vi "genIOL_Aligning.vi"(0 "Iris path":path=path "D:/IRISSoft LV2016 beta/Host Demo/ThorlabsData/Eye1/VSCAN_0002.raw", 1 "endJ5":dbl=30000.0, 2 "PC path":path=path "D:/IRISSoft LV2016 beta/Host Demo/ThorlabsData/Eye1/VSCAN_0003.raw", 3 "endPt":dbl[](array[numeric]), 4 "Distance from incision":dbl=1.0, 5 "OCT offset":dbl=13.0) -> (6 "Align_traj":dbl[][](array[numeric]), 7 "Inject_traj":dbl[][](array[numeric]), 8 "Whole_traj":dbl[][](array[numeric]))   [LabVIEW 2016]
uses:
  <vilib>/Math Plots/3D Math Plots/3D Scatter/3D Scatter XCtrl/3D Scatter.xctl
  Subsystems/Global Variables.vi
  <vilib>/Utility/file.llb/Write Delimited Spreadsheet (DBL).vi
  <vilib>/Math Plots/3D Math Plots/3D Scatter/3D Scatter Datatype/Public/Plot Helper (Vector).vi
  <vilib>/Analysis/NI_AALBase.lvlib
  <vilib>/Analysis/1siggen.llb/Ramp Pattern by Samples.vi
  <vilib>/gmath/NI_Gmath.lvlib
  <vilib>/Math Plots/3D Math Plots/3D Scatter/3D Scatter Datatype/3D Scatter Datatype.lvclass
  <vilib>/Math Plots/3D Math Plots/3D Plot/3D Plot Datatype/3D Plot Datatype.lvclass
panel:
  out "Actual Injection Plot 2":refnum<class "3D Plot Datatype.lvclass">[](xcontrol)
  out "current loop # 3":dbl
  out "Actual joint angles":dbl[][](array[numeric])
  out "Planned joint angles":dbl[][](array[numeric])
  out "Planned injection":dbl[][](array[numeric])
  out "Incision point index 3":dbl
  out "Incision point index 2":dbl
  out "Error in operational space":dbl[][](graph)
  out "current loop # 2":dbl
  out "time":dbl[](array[numeric])
  out "incision":dbl[](array[numeric])
  out "traj operational space":dbl[][](array[numeric])
  out "Incision point":dbl[](array[numeric])
  out "Implement Injection Plot":refnum<class "3D Plot Datatype.lvclass">[](xcontrol)
  out "Implement joint angles":dbl[][](graph)
  out "min dist":dbl
  out "Actual Injection Plot":refnum<class "3D Plot Datatype.lvclass">[](xcontrol)
  out "End manual joint":dbl[](array[numeric])
  out "Start manual joint":dbl[](array[numeric])
  out "Planed joint angles":dbl[][](graph)
  out "Actual joint angles":dbl[][](graph)
  out "traj":dbl[][](array[numeric])
  out "max dist":dbl
  out "Offset":dbl[][](array[numeric])
  out "Incision point index":dbl
  out "Planed Injection Plot":refnum<class "3D Plot Datatype.lvclass">[](xcontrol)
  out "current loop #":dbl
  out "x coordinates size 3":dbl
  out "x coordinates size 2":dbl
  out "x coordinates size":dbl
  out "x coordinates":dbl[](array[numeric])
  out "z coordinates":dbl[](array[numeric]) format="%#_13g"
  out "y coordinates":dbl[](array[numeric]) format="%#_13g"
  out "x coodi 2nd":dbl[](array[numeric]) format="%#_13g"
  in  "Total Time":dbl=60.0
  in  "Arm ID Ind":i32
  in  "Tip out Posit":dbl[](array[numeric])=[0.0, 0.0, 0.0] caption="Position [mm]" format="%#.3f"
  in  "Cycle Time [sec]":dbl[](array[numeric])=[60.0, 90.0, 120.0]
  out "zVisTraj":dbl[](array[numeric]) format="%_6g"
  out "yVisTraj":dbl[](array[numeric]) format="%_6g"
  out "xVisTraj":dbl[](array[numeric]) format="%_6g"
  in  "Sampling Rate [Hz]":i32=1000
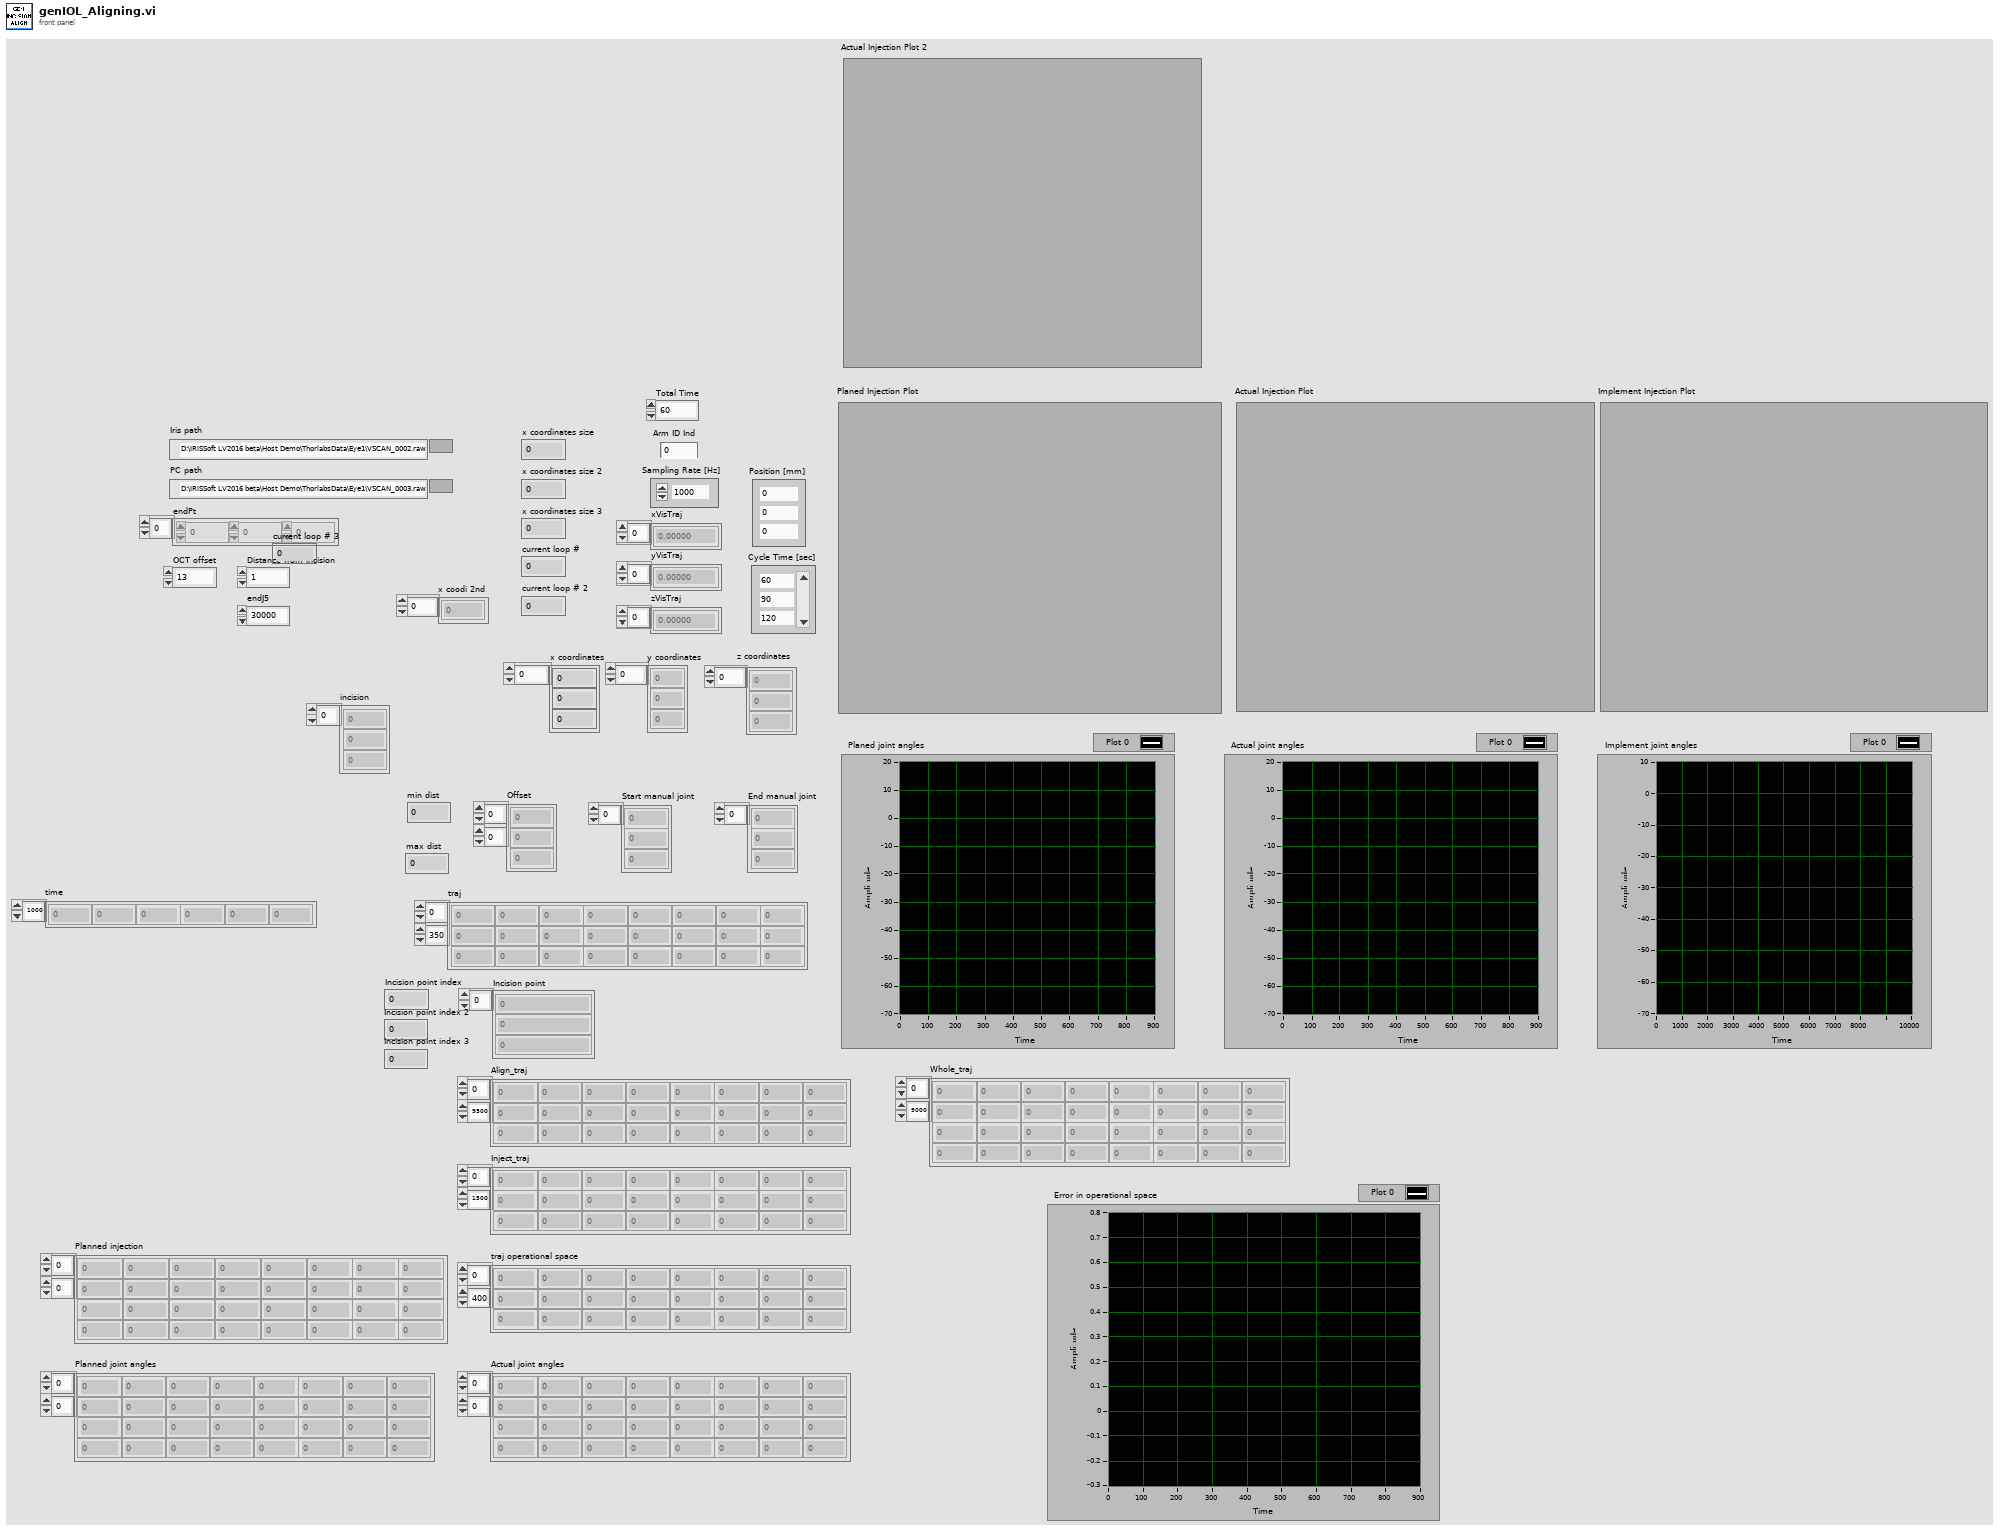
[diagram p1: front panel]
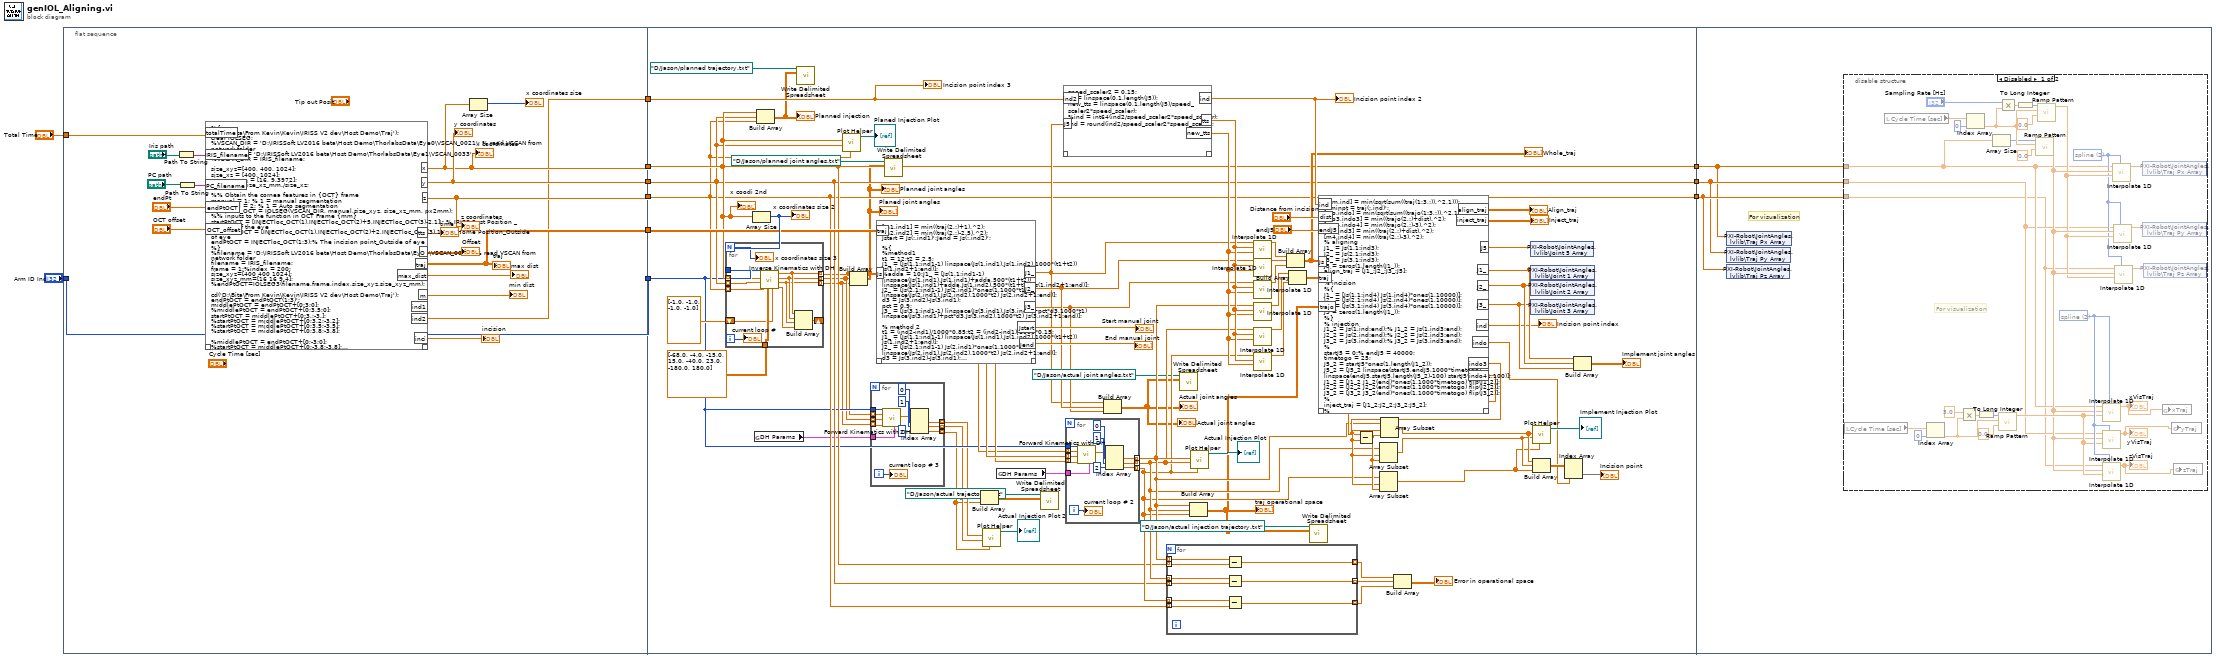
[diagram p0: block diagram]
diagram:
  n1 = flat-sequence {
    tunnel: "Arm ID Ind" -> [w30]
    tunnel: [w30] -> w10
    tunnel: [w26] -> w6
    tunnel: [w28] -> w5
    tunnel: [w27] -> w4
    tunnel: "Total Time" -> [w29]
    tunnel: [w13] -> w2
    tunnel: [w12] -> w1
    tunnel: w10 -> [w39]
    tunnel: [w52] -> w9
    tunnel: [w51] -> w8
    tunnel: [w50] -> w7
    tunnel: w6 -> [w52]
    tunnel: w5 -> [w51]
    tunnel: w4 -> [w50]
    tunnel: w2 -> [w63]
    tunnel: w1 -> [w54]
    tunnel: w9 -> [w152]
    tunnel: w8 -> [w153]
    tunnel: w7 -> [w154]
    frame #0 {
      n2 = Path To String(path="Iris path") -> (string=w20:string)
      n3 = Path To String(path="PC path") -> (string=w21:string)
      n4 = script code="%{\ncd('D:\\Bita\\From Kevin\\Kevin\\IRISS V2 dev\\Host Demo\\Traj');\nclear IOLSEG;\n%VSCAN_DIR = 'D:\\IRISSoft LV2016 beta\\Host Demo\\ThorlabsData\\Eye0\\VSCAN_0021'; % read VSCAN from network folder \nVSCAN_DIR = 'D:\\IRISSoft LV2016 beta\\Host Demo\\ThorlabsData\\Eye1\\VSCAN_0033';\n%VSCAN_DIR = IRIS_filename;\n\nsize_xyz=[400, 400, 1024];\nsize_xz = [400, 1024]; \nsize_xz_mm = [16, 9.3972]; \npx2mm = size_xz_mm./size_xz; \n    \n%% Obtain the cornea features in {OCT} frame\nmanual = 1; % 1 = manual segmentation\n%manual = 2; % 1 = Auto segmentation\nINJECTloc_OCT = IOLSEG(VSCAN_DIR, manual,size_xyz, size_xz_mm, px2mm);\n%% inputs to the function in OCT Frame {mm}\nstartPtOCT = [INJECTloc_OCT(1),INJECTloc_OCT(2)+5,INJECTloc_OCT(3)-2,1]'; % IRISS Rest Position _Outside of the eye\nmiddlePtOCT = [INJECTloc_OCT(1),INJECTloc_OCT(2)+2,INJECTloc_OCT(3),1]'; % Home Position_Outside of eye\nendPtOCT = INJECTloc_OCT(1:3);% The incision point_Outside of eye\n%}\n%filename = 'D:\\IRISSoft LV2016 beta\\Host Demo\\ThorlabsData\\Eye0\\VSCAN_0021'; % read VSCAN from network folder \nfilename = IRIS_filename;\nframe = 1;%index = 200;\nsize_xyz=[400 400 1024];\nsize_xyz_mm=[16 16 9.4];\n%endPtOCT=IOLSEG3(filename,frame,index,size_xyz,size_xyz_mm);\n\ncd('D:\\Bita\\From Kevin\\Kevin\\IRISS V2 dev\\Host Demo\\Traj');\nendPtOCT = endPtOCT(1:3)';\nmiddlePtOCT = endPtOCT+[0;3;0];\n%middlePtOCT = endPtOCT+[0;3.5;0];\nstartPtOCT = middlePtOCT+[0;3.;-3.];\n%startPtOCT = middlePtOCT+[0;3.2;-3.2];\n%startPtOCT = middlePtOCT+[0;3.5;-3.5];\n%startPtOCT = middlePtOCT+[0;3.8;-3.8];\n\n%middlePtOCT = endPtOCT+[0;-3;0];\n%startPtOCT = middlePtOCT+[0;-3.8;-3.8];\n\n%IRIS_filename = 'D:\\IRISSoft LV2016 beta\\Host Demo\\ThorlabsData\\Eye0\\VSCAN_0021.raw';\n%PC_filename = 'D:\\IRISSoft LV2016 beta\\Host Demo\\ThorlabsData\\Eye0\\VSCAN_0022.raw';\n%OCT_offset = 7; %OCT_offset = 0;\n%IRIS_filename = 'D:\\IRISSoft LV2016 beta\\Host Demo\\ThorlabsData\\Eye1\\VSCAN_0002.raw';\n%PC_filename = 'D:\\IRISSoft LV2016 beta\\Host Demo\\ThorlabsData\\Eye1\\VSCAN_0003.raw';\n%OCT_offset = 13;\n%speed_scaler = 0.15;\nspeed_scaler = 5;\n[tts,traj2,ind1,ind2]=IOL_injection_trajectory(startPtOCT,middlePtOCT,endPtOCT,IRIS_filename,PC_filename,OCT_offset,speed_scaler);\nTOI_file= 'D:\\IRISSoft LV2016 beta\\Host Demo\\TOI_static'\nfid_TOI = fopen(TOI_file,'r');\nTOI=fscanf(fid_TOI,'%f');\nTOI= reshape(TOI, [4 4])';\nfclose(fid_TOI);\n\nmax_dist = max(sqrt(sum(diff(traj2,1,2).^2,1)));\nO = inv(TOI)*[endPtOCT(1)-3;endPtOCT(2)-3;endPtOCT(3);1];\n%O = inv(TOI)*[endPtOCT(1);endPtOCT(2);endPtOCT(3);1];\n%{\ninit_X = 40;init_Y = 55;init_Z = 100;\ntime_to_go = norm(O(1:3))/.5;\nstage_X = linspace(init_X,init_X+O(1),1000*time_to_go);\nstage_Y = linspace(init_Y,init_Y+O(2),1000*time_to_go);\nstage_Z = linspace(init_Z,init_Z+O(3),1000*time_to_go);\n%}\n\nTOI2 = inv(TOI);TOI2(1:3,4) = TOI2(1:3,4)-O(1:3);\n%traj = inv(TOI)*[traj2;ones(1,size(traj2,2))]-O;\n%traj = TOI2*[traj2;ones(1,size(traj2,2))];\ntraj = inv(TOI)*[traj2(1,:)-3;traj2(2,:)-3;traj2(3,:);ones(1,size(traj2,2))]-O;\n%{\nTOI2_file= 'D:\\IRISSoft LV2016 beta\\Host Demo\\new_TOI.txt'\nfid_TOI2 = fopen(TOI2_file,'r');\nTOI2=fscanf(fid_TOI2,'%f');\nTOI2= reshape(TOI2, [4 4]);\nfclose(fid_TOI2);\ntraj = inv(TOI2)*[traj2;ones(1,size(traj2,2))];\n%}\n\nx = traj(1,:);y = traj(2,:);z = traj(3,:);\n[m,ind] = min(sqrt(sum((traj(1:3,:)).^2,1)));\ninci = traj(:,ind)';"("totalTime"=w29, "IRIS_filename"=w20, "PC_filename"=w21, "endPtOCT"="endPt", "OCT_offset"="OCT offset") -> ("x"=w26:dbl[], "y"=w28:dbl[], "z"=w27:dbl[], "O"=→"Offset":dbl[][], "max_dist"=→"max dist":dbl, "traj"=w13:dbl[][], "ind2"=w12:dbl, "m"=→"min dist":dbl, "inci"=→"incision":dbl[], "tts"=→"time":dbl[])  [unwired: 1 in, 2 out]
      "y coordinates" <- w28
      "z coordinates" <- w27
      "x coordinates" <- w26
      "traj" <- w13
      n5 = Array Size(array=w26) -> (size(s)=→"x coordinates size":i32)
    }
    frame #1 {
      n6 = Array Size(array=w52) -> (size(s)=w103:i32)
      "x coordinates size 2" <- w103
      n7 = for {
        N: w103 -> [w151]
        tunnel: w39 -> [w148]
        tunnel: w52 -> [w147] mode=indexing
        tunnel: w51 -> [w146] mode=indexing
        tunnel: w50 -> [w145] mode=indexing
        tunnel: [w140] -> w37 mode=indexing
        tunnel: [w141] -> w38 mode=indexing
        tunnel: [w139] -> w36 mode=indexing
        tunnel: dbl[][] [[-68.0, -4.0], [-15.0, 15.0], [-40.0, 23.0], [-180.0, 180.0]] ("Joint Limits") -> [w144]
        shift-right: [w149] -> _
        shift-left: dbl[] [-1.0, -1.0, -1.0, -1.0] ("Initial guess") -> [w143]
        i -> [w150]
        n8 = call "Inverse Kinematics with DH.vi"("Initial guess"=w143, "Joint Limits"=w144, "armID"=w148, "z"=w145, "y"=w146, "x"=w147) -> ("j4"=w142:dbl, "j3"=w139:dbl, "j2"=w140:dbl, "j1"=w141:dbl)  [unwired: 2 in]
        n9 = Build Array(w141, w140, w139, w142) -> (w149:dbl[])
        "x coordinates size 3" <- w151
        "current loop #" <- w150
      }
      n10 = global read "Global Variables.vi" "DH Params"() -> (w41:cluster{"d_DH":dbl[][], "ty":dbl[][]})
      n11 = Build Array(w52, w51, w50) -> (w49:dbl[][])
      "Planned injection" <- w49
      n12 = call-poly <vilib>:"Write Delimited Spreadsheet.vi"("file path (dialog if empty)"=path "D:/Jason/planned trajectory.txt", "2D data"=w49) -> ()  [unwired: 12 in, 2 out]
      n13 = call-poly <vilib>:"Plot Helper.vi"("z vector"=w50, "y vector"=w51, "x vector"=w52) -> ("3D Plot lvclass Array out"=→"Planed Injection Plot":refnum<class "3D Plot Datatype.lvclass">[])  [unwired: 3 in, 5 out]
      n14 = Build Array(w38, w37, w36) -> (w46:dbl[][])
      "Planed joint angles" <- w46
      "Planned joint angles" <- w46
      n15 = for {
        tunnel: w39 -> [w109]
        tunnel: w38 -> [w110] mode=indexing
        tunnel: w37 -> [w108] mode=indexing
        tunnel: w36 -> [w107] mode=indexing
        tunnel: [w113] -> w35 mode=indexing
        tunnel: [w112] -> w34 mode=indexing
        tunnel: [w111] -> w33 mode=indexing
        tunnel: w41 -> [w105]
        i -> [w104]
        n16 = call "Forward Kinematics with DH.vi"("DH Params"=w105, "j3"=w107, "j2"=w108, "j1"=w110, "armID"=w109) -> ("XYZ With DH Calibration"=w106:dbl[])  [unwired: 6 in]
        n17 = Index Array(array=w106, index #1=0 ("index"), index #2=1 ("index"), index #3=2 ("index")) -> (element #1=w113:dbl, element #2=w112:dbl, element #3=w111:dbl)
        "current loop # 3" <- w104
      }
      n18 = script code="[m1,ind1] = min((traj(2,:)+1).^2);\n[m2,ind2] = min((traj(2,:)-2.5).^2);\nJstart = Js(:,ind1)';Jend = Js(:,ind2)';\n\n%{\n%method1\nt1 = 12;t2 = 2.5;\nJ1_ = [Js(1,1:ind1-1) linspace(Js(1,ind1),Js(1,ind2),1000*(t1+t2)) Js(1,ind2+1:end)];\n%adda = 10;J1_ = [Js(1,1:ind1-1) linspace(Js(1,ind1),Js(1,ind1)+adda,500*(t1+t2)) linspace(Js(1,ind1)+adda,Js(1,ind2),500*(t1+t2)) Js(1,ind2+1:end)];\nJ2_ = [Js(2,1:ind1-1) Js(2,ind1)*ones(1,1000*t1) linspace(Js(2,ind1),Js(2,ind2),1000*t2) Js(2,ind2+1:end)];\nd3 = Js(3,ind2)-Js(3,ind1);\npct = 0.9;\nJ3_ = [Js(3,1:ind1-1) linspace(Js(3,ind1),Js(3,ind1)+pct*d3,1000*t1) linspace(Js(3,ind1)+pct*d3,Js(3,ind2),1000*t2) Js(3,ind2+1:end)];\n\n% method 2\nt1 = (ind2-ind1)/1000*0.85;t2 = (ind2-ind1)/1000*0.15;\nJ1_ = [Js(1,1:ind1-1) linspace(Js(1,ind1),Js(1,ind2),1000*(t1+t2)) Js(1,ind2+1:end)];\nJ2_ = [Js(2,1:ind1-1) Js(2,ind1)*ones(1,1000*t1) linspace(Js(2,ind1),Js(2,ind2),1000*t2) Js(2,ind2+1:end)];\nd3 = Js(3,ind2)-Js(3,ind1);\npct = 0.9;\nJ3_ = [Js(3,1:ind1-1) linspace(Js(3,ind1),Js(3,ind1)+pct*d3,1000*t1) linspace(Js(3,ind1)+pct*d3,Js(3,ind2),1000*t2) Js(3,ind2+1:end)];\n%}\nJ1_ = [Js(1,1:ind1-1) linspace(Js(1,ind1),Js(1,ind2),ind2-ind1+1) Js(1,ind2+1:end)];\nJ2_ = [Js(2,1:ind1-1) linspace(Js(2,ind1),Js(2,ind2),ind2-ind1+1) Js(2,ind2+1:end)];\nJ3_ = [Js(3,1:ind1-1) linspace(Js(3,ind1),Js(3,ind2),ind2-ind1+1) Js(3,ind2+1:end)];"("Js"=w46, "traj"=w63) -> ("J1_"=w68:dbl[], "J2_"=w91:dbl[], "J3_"=w90:dbl[], "Jstart"=→"Start manual joint":dbl[], "Jend"=→"End manual joint":dbl[])  [unwired: 1 in, 1 out]
      n19 = call-poly <vilib>:"Write Delimited Spreadsheet.vi"("file path (dialog if empty)"=path "D:/Jason/planned joint angles.txt", "2D data"=w46) -> ()  [unwired: 12 in, 2 out]
      n20 = Build Array(w35, w34, w33) -> (w32:dbl[][])
      n21 = call-poly <vilib>:"Plot Helper.vi"("z vector"=w33, "y vector"=w34, "x vector"=w35) -> ("3D Plot lvclass Array out"=→"Actual Injection Plot 2":refnum<class "3D Plot Datatype.lvclass">[])  [unwired: 3 in, 5 out]
      n22 = global read "Global Variables.vi" "DH Params"() -> (w95:cluster{"d_DH":dbl[][], "ty":dbl[][]})
      n23 = call-poly <vilib>:"Write Delimited Spreadsheet.vi"("file path (dialog if empty)"=path "D:/Jason/actual trajectory2.txt", "2D data"=w32) -> ()  [unwired: 12 in, 2 out]
      n24 = script code="speed_scaler2 = 0.15;\ntts = linspace(0,1,length(J5));\nnew_tts = linspace(0,1,length(J5)/speed_scaler2*speed_scaler);\n%ind = int64(ind2/speed_scaler2*speed_scaler);\nind = round(ind2/speed_scaler2*speed_scaler);"("J5"=w68, "ind2"=w54) -> ("new_tts"=w92:dbl[], "tts"=w93:dbl[], "ind"=w55:dbl)  [unwired: 1 in, 1 out]
      "Incision point index 2" <- w55
      n25 = for {
        tunnel: w39 -> [w131]
        tunnel: w68 -> [w132] mode=indexing
        tunnel: w91 -> [w130] mode=indexing
        tunnel: w90 -> [w129] mode=indexing
        tunnel: [w135] -> w62 mode=indexing
        tunnel: [w134] -> w61 mode=indexing
        tunnel: [w133] -> w60 mode=indexing
        tunnel: w95 -> [w127]
        i -> [w126]
        n26 = call "Forward Kinematics with DH.vi"("DH Params"=w127, "j3"=w129, "j2"=w130, "j1"=w132, "armID"=w131) -> ("XYZ With DH Calibration"=w128:dbl[])  [unwired: 6 in]
        n27 = Index Array(array=w128, index #1=0 ("index"), index #2=1 ("index"), index #3=2 ("index")) -> (element #1=w135:dbl, element #2=w134:dbl, element #3=w133:dbl)
        "current loop # 2" <- w126
      }
      n28 = Build Array(w68, w91, w90) -> (w44:dbl[][])
      "Actual joint angles" <- w44
      "Actual joint angles" <- w44
      n29 = for {
        tunnel: w52 -> [w122] mode=indexing
        tunnel: w51 -> [w123] mode=indexing
        tunnel: w50 -> [w120] mode=indexing
        tunnel: w62 -> [w125] mode=indexing
        tunnel: w61 -> [w124] mode=indexing
        tunnel: w60 -> [w121] mode=indexing
        tunnel: [w119] -> w58 mode=indexing
        tunnel: [w118] -> w57 mode=indexing
        tunnel: [w117] -> w56 mode=indexing
        n30 = Subtract(x=w125, y=w122) -> (x-y=w119:dbl)
        n31 = Subtract(x=w124, y=w123) -> (x-y=w118:dbl)
        n32 = Subtract(x=w121, y=w120) -> (x-y=w117:dbl)
      }
      n33 = call-poly <vilib>:"Write Delimited Spreadsheet.vi"("file path (dialog if empty)"=path "D:/Jason/actual joint angles.txt", "2D data"=w44) -> ()  [unwired: 12 in, 2 out]
      n34 = Build Array(w62, w61, w60) -> (w42:dbl[][])
      "traj operational space" <- w42
      n35 = call-poly <vilib>:"Plot Helper.vi"("z vector"=w60, "y vector"=w61, "x vector"=w62) -> ("3D Plot lvclass Array out"=→"Actual Injection Plot":refnum<class "3D Plot Datatype.lvclass">[])  [unwired: 3 in, 5 out]
      n36 = call <vilib>:"Interpolate 1D.vi"("xi"=w92, "X"=w93, "Y"=w68) -> ("yi"=w89:dbl[])  [unwired: 6 in, 2 out]
      n37 = call <vilib>:"Interpolate 1D.vi"("xi"=w92, "X"=w93, "Y"=w91) -> ("yi"=w88:dbl[])  [unwired: 6 in, 2 out]
      n38 = call <vilib>:"Interpolate 1D.vi"("xi"=w92, "X"=w93, "Y"=w90) -> ("yi"=w87:dbl[])  [unwired: 6 in, 2 out]
      n39 = call <vilib>:"Interpolate 1D.vi"("xi"=w92, "X"=w93, "Y"=w62) -> ("yi"=w85:dbl[])  [unwired: 6 in, 2 out]
      n40 = call <vilib>:"Interpolate 1D.vi"("xi"=w92, "X"=w93, "Y"=w61) -> ("yi"=w83:dbl[])  [unwired: 6 in, 2 out]
      n41 = call <vilib>:"Interpolate 1D.vi"("xi"=w92, "X"=w93, "Y"=w60) -> ("yi"=w84:dbl[])  [unwired: 6 in, 2 out]
      n42 = Build Array(w89, w88, w87) -> (w53:dbl[][])
      "Whole_traj" <- w53
      n43 = Build Array(w85, w83, w84) -> (w86:dbl[][])
      n44 = call-poly <vilib>:"Write Delimited Spreadsheet.vi"("file path (dialog if empty)"=path "D:/Jason/actual injection trajectory.txt", "2D data"=w42) -> ()  [unwired: 12 in, 2 out]
      n45 = script code="%[m,ind] = min(sqrt(sum((traj(1:3,:)).^2,1)));\n%minpt = traj(:,ind)';\n[mo,indo] = min(sqrt(sum((trajo(1:3,:)).^2,1)));\n[mo3,indo3] = min((trajo(2,:)+dist).^2);\n[mo4,indo4] = min((trajo(2,:)-3).^2);\n[m3,ind3] = min((traj(2,:)+dist).^2);\n[m4,ind4] = min((traj(2,:)-3).^2);\n% aligning\nJ1_ = Js(1,1:ind3);\nJ2_ = Js(2,1:ind3);\nJ3_ = Js(3,1:ind3);\nJ5 = zeros(1,length(J1_));\nalign_traj = [J1_;J2_;J3_;J5];\n%\n% incision\n%{\nJ1_ = [Js(1,1:ind4) Js(1,ind4)*ones(1,10000)];\nJ2_ = [Js(2,1:ind4) Js(2,ind4)*ones(1,10000)];\nJ3_ = [Js(3,1:ind4) Js(3,ind4)*ones(1,10000)];\nJ5 = zeros(1,length(J1_));\n%}\n% injection\nJ1_2 = Js(1,ind:end);% J1_2 = Js(1,ind3:end);\nJ2_2 = Js(2,ind:end);% J2_2 = Js(2,ind3:end);\nJ3_2 = Js(3,ind:end);% J3_2 = Js(3,ind3:end);\n%\nstartJ5 = 0;% endJ5 = 40000;\ntimetogo = 25;\nJ5_2 = startJ5*ones(1,length(J1_2));\nJ5_2 = [J5_2 linspace(startJ5,endJ5,1000*timetogo) linspace(endJ5,startJ5,length(J5_2)-100) startJ5*ones(1,100)];\nJ1_2 = [J1_2 J1_2(end)*ones(1,1000*timetogo) flip(J1_2)];\nJ2_2 = [J2_2 J2_2(end)*ones(1,1000*timetogo) flip(J2_2)];\nJ3_2 = [J3_2 J3_2(end)*ones(1,1000*timetogo) flip(J3_2)];\n%\ninject_traj = [J1_2;J2_2;J3_2;J5_2];\n%"("Js"=w53, "traj"=w86, "dist"="Distance from incision", "endJ5"="endJ5", "trajo"=w42, "ind"=w55) -> ("J1_"=w77:dbl[], "J2_"=w76:dbl[], "J3_"=w75:dbl[], "ind"=→"Incision point index":dbl, "J5"=w78:dbl[], "align_traj"=→"Align_traj":dbl[][], "inject_traj"=→"Inject_traj":dbl[][], "indo3"=w67:dbl, "indo4"=w66:dbl, "indo"=w69:dbl)  [unwired: 1 in, 1 out]
      n46 = Subtract(x=w66, y=w67) -> (x-y=w73:dbl)
      n47 = Array Subset(array=w60, index=w67, length=w73) -> (w70:dbl[])
      n48 = Array Subset(array=w61, index=w67, length=w73) -> (w71:dbl[])
      n49 = Array Subset(array=w62, index=w67, length=w73) -> (w72:dbl[])
      n50 = Build Array(w58, w57, w56) -> (→"Error in operational space":dbl[][])
      n51 = shared-variable "PXI-Robot\\JointAngles.lvlib\\Joint 5 Array"(w78) -> ()  [unwired: 1 in, 1 out]
      n52 = shared-variable "PXI-Robot\\JointAngles.lvlib\\Joint 1 Array"(w77) -> ()  [unwired: 1 in, 1 out]
      n53 = shared-variable "PXI-Robot\\JointAngles.lvlib\\Joint 2 Array"(w76) -> ()  [unwired: 1 in, 1 out]
      n54 = shared-variable "PXI-Robot\\JointAngles.lvlib\\Joint 3 Array"(w75) -> ()  [unwired: 1 in, 1 out]
      n55 = call-poly <vilib>:"Plot Helper.vi"("z vector"=w70, "y vector"=w71, "x vector"=w72) -> ("3D Plot lvclass Array out"=→"Implement Injection Plot":refnum<class "3D Plot Datatype.lvclass">[])  [unwired: 3 in, 5 out]
      n56 = Build Array(w72, w71, w70) -> (w97:dbl[][])
      n57 = Index Array(array=w97, index (col)=w69) -> (element=→"Incision point":dbl[])  [unwired: 1 in]
      n58 = Build Array(w77, w76, w75) -> (→"Implement joint angles":dbl[][])
      "x coodi 2nd" <- w52
      "Incision point index 3" <- w54
    }
    frame #2 {
      # "For visualization"
      n59 = shared-variable "PXI-Robot\\JointAngles.lvlib\\Traj Py Array"(w153) -> ()  [unwired: 1 in, 1 out]
      n60 = shared-variable "PXI-Robot\\JointAngles.lvlib\\Traj Pz Array"(w154) -> ()  [unwired: 1 in, 1 out]
      n61 = shared-variable "PXI-Robot\\JointAngles.lvlib\\Traj Px Array"(w152) -> ()  [unwired: 1 in, 1 out]
      n62 = disable-structure shown="Disabled" {
        disable-tunnel: w152 -> [w160 _]
        disable-tunnel: w153 -> [w159 _]
        disable-tunnel: w154 -> [w158 _]
        frame Disabled {
          w172 = 2 items=["nearest", "linear", "spline", "cubic Hermite", "Lagrange"] ("method")
          w161 = 2 items=["nearest", "linear", "spline", "cubic Hermite", "Lagrange"] ("method")
          # "For visualization"
          n63 = local read "Cycle Time [sec]"() -> (w166:dbl[])
          n64 = local read "Cycle Time [sec]"() -> (w184:dbl[])
          n65 = Index Array(array=w166, index=0) -> (element=w167:dbl)
          n66 = Multiply(x=5.0, y=w167) -> (x*y=w169:dbl)
          n67 = Index Array(array=w184, index=0) -> (element=w177:dbl)
          n68 = To Long Integer(number=w169) -> (32bit integer=w170:i32)
          n69 = Array Size(array=w160) -> (size(s)=w176:i32)
          n70 = call-poly <vilib>:"Ramp Pattern.vi"("start"=0.0, "end"=w167, "samples"=w170) -> ("Ramp Pattern"=w164:dbl[])  [unwired: 7 in, 1 out]
          n71 = Multiply(x="Sampling Rate [Hz]", y=w177) -> (x*y=w180:dbl)
          n72 = To Long Integer(number=w180) -> (32bit integer=w181:i32)
          n73 = call-poly <vilib>:"Ramp Pattern.vi"("start"=0.0, "end"=w177, "samples"=w176) -> ("Ramp Pattern"=w163:dbl[])  [unwired: 7 in, 1 out]
          n74 = call-poly <vilib>:"Ramp Pattern.vi"("start"=0.0, "end"=w177, "samples"=w181) -> ("Ramp Pattern"=w162:dbl[])  [unwired: 7 in, 1 out]
          n75 = call <vilib>:"Interpolate 1D.vi"("method"=w172, "xi"=w164, "X"=w163, "Y"=w160) -> ("yi"=w155:dbl[])  [unwired: 5 in, 2 out]
          "xVisTraj" <- w155
          n76 = call <vilib>:"Interpolate 1D.vi"("method"=w172, "xi"=w164, "X"=w163, "Y"=w159) -> ("yi"=w156:dbl[])  [unwired: 5 in, 2 out]
          "yVisTraj" <- w156
          n77 = call <vilib>:"Interpolate 1D.vi"("method"=w172, "xi"=w164, "X"=w163, "Y"=w158) -> ("yi"=w157:dbl[])  [unwired: 5 in, 2 out]
          "zVisTraj" <- w157
          n78 = call <vilib>:"Interpolate 1D.vi"("method"=w161, "xi"=w162, "X"=w163, "Y"=w160) -> ("yi"=w174:dbl[])  [unwired: 5 in, 2 out]
          n79 = call <vilib>:"Interpolate 1D.vi"("method"=w161, "xi"=w162, "X"=w163, "Y"=w159) -> ("yi"=w175:dbl[])  [unwired: 5 in, 2 out]
          n80 = call <vilib>:"Interpolate 1D.vi"("method"=w161, "xi"=w162, "X"=w163, "Y"=w158) -> ("yi"=w173:dbl[])  [unwired: 5 in, 2 out]
          n81 = shared-variable "PXI-Robot\\JointAngles.lvlib\\Traj Px Array"(w174) -> ()  [unwired: 1 in, 1 out]
          n82 = shared-variable "PXI-Robot\\JointAngles.lvlib\\Traj Py Array"(w175) -> ()  [unwired: 1 in, 1 out]
          n83 = shared-variable "PXI-Robot\\JointAngles.lvlib\\Traj Pz Array"(w173) -> ()  [unwired: 1 in, 1 out]
          n84 = global write "Global Variables.vi" "xTraj"(w155) -> ()
          n85 = global write "Global Variables.vi" "yTraj"(w156) -> ()
          n86 = global write "Global Variables.vi" "zTraj"(w157) -> ()
        }
        frame Enabled {
        }
      }
    }
  }
